vi "Abort.vi"(8 "error in (no error)":errorcluster, 11 "PIPXI40 Base in":refnum<class "PIPX40 Base.lvclass">) -> (0 "error out":errorcluster, 3 "PIPXI40 Base out":refnum<class "PIPX40 Base.lvclass">)   [LabVIEW 2020, in "Pickering.lvlib" / "PIPX40 Base.lvclass"]
uses:
  PIPX40 Base.lvclass
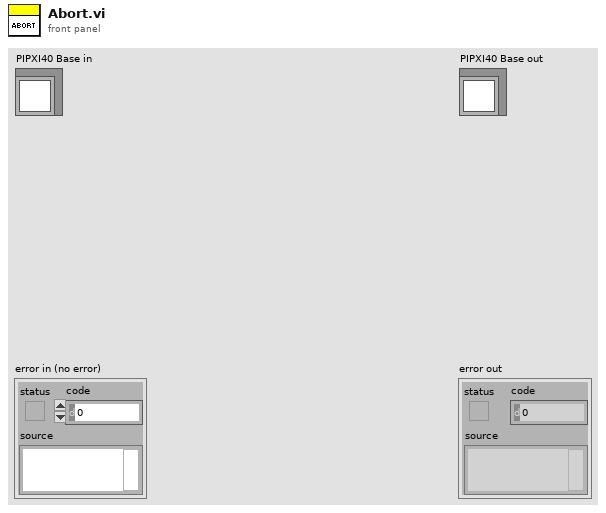
[diagram p1: front panel]
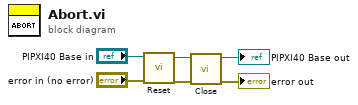
[diagram p0: block diagram]
diagram:
  n1 = call-dynamic "Reset.vi"("error in (no error)"="error in (no error)", "PIPXI40 Base in"="PIPXI40 Base in") -> ("error out"=w5:errorcluster, "PIPXI40 Base out"=w6:refnum<class "PIPX40 Base.lvclass">)  [unwired: 8 in]
  n2 = call-dynamic "Close.vi"("error in (no error)"=w5, "PIPXI40 Base in"=w6) -> ("error out"=→"error out":errorcluster, "PIPXI40 Base out"=→"PIPXI40 Base out":refnum<class "PIPX40 Base.lvclass">)  [unwired: 8 in]
